vi "SLSC Get Items from Tree Control.vi"(11 "Item":T1) -> (1 "Value":string, 2 "Datatype":string, 3 "Type of Channel":string, 4 "Enum Type":string, 5 "Reset Value":string)   [LabVIEW 2019, in "SLSC Tree Control.lvlib"]
doc: "Separates each element of the tree item."
uses:
  SLSC Tree Control.lvlib
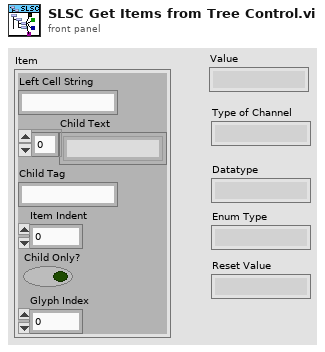
[diagram p1: front panel]
types:
  T1 = cluster{"Left Cell String":string, "Child Text":string[], "Child Tag":string, "Item Indent":i32, "Child Only?":bool, "Glyph Index":i32}
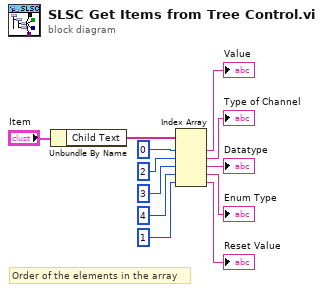
[diagram p0: block diagram]
diagram:
  # "Order of the elements in the array"
  n1 = Unbundle By Name("Item") -> ("Child Text"=w10:string[])
  n2 = Index Array(array=w10, index #1=0 ("index"), index #2=2 ("index"), index #3=3 ("index"), index #4=4 ("index"), index #5=1 ("index")) -> (element #1=→"Value":string, element #2=→"Type of Channel":string, element #3=→"Datatype":string, element #4=→"Enum Type":string, element #5=→"Reset Value":string)
